vi "calculateRobotModelProgress.vi"(5 "current state":i32, 7 "start":bool, 10 "totalNumerOfTests":dbl) -> (2 "progress":dbl)   [LabVIEW 2021, in "Game.lvclass"]
uses:
  Game.lvclass
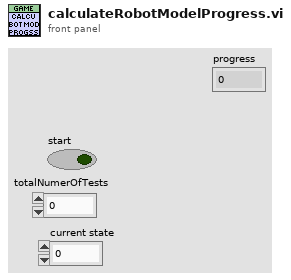
[diagram p1: front panel]
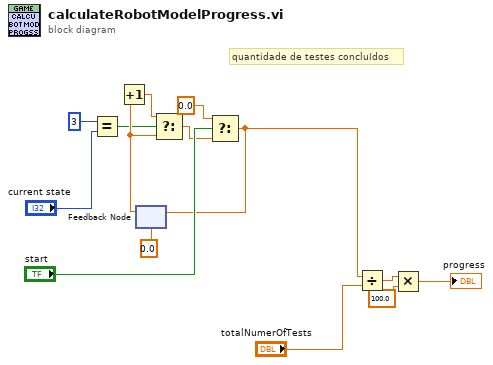
[diagram p0: block diagram]
diagram:
  # "quantidade de testes concluídos"
  n1 = Equal?(x=3, y="current state") -> (x = y?=w10:bool)
  n2 = feedback #1(0.0) -> (w13:dbl)
  n3 = Increment(x=w13) -> (x+1=w11:dbl)
  n4 = Select(t=w11, s=w10, f=w13) -> (s? t:f=w5:dbl)
  n5 = Select(t=0.0, s="start", f=w5) -> (s? t:f=w3:dbl)
  n6 = feedback-in #1(w3) -> ()
  n7 = Divide(x=w3, y="totalNumerOfTests") -> (x/y=w2:dbl)
  n8 = Multiply(x=w2, y=100.0) -> (x*y=→"progress":dbl)
